vi "GetThermAlarmAnalogInputUnitsValue.vi"(8 "error in":errorcluster, 10 "ThermAlarm number":T1=1 items=["ThermAlarm 1"=1, "ThermAlarm 2"=2, "ThermAlarm 3"=3, "ThermAlarm 4"=4], 11 "VISA resource name":refnum<visa-resource-name>) -> (0 "error out":errorcluster, 2 "ThermAlarm analog input units value":string, 3 "VISA resource name out":refnum<visa-resource-name>)   [LabVIEW 2023, in "Thermotron 8800.lvlib"]
doc: "AACH\nCommand name: Therm-Alarm analog input value\nCommand name: Send Therm-Alarm analog input units value\nCommand type: System status\nDescription: The 8800 returns 1-3 characters for the value. Common unit codes are % and T (torr).\nSyntax: AACHn?\nWhere n is a Therm-Alarm number (1 to 4).\nData type: 1-3 characters\nQuery example: AACH1?\n8800 response: T (The analog input of Therm-Alarm 1 is programmed in torr.)"
uses:
  Thermotron 8800.lvlib
  Private/ThermAlarmNumber.ctl
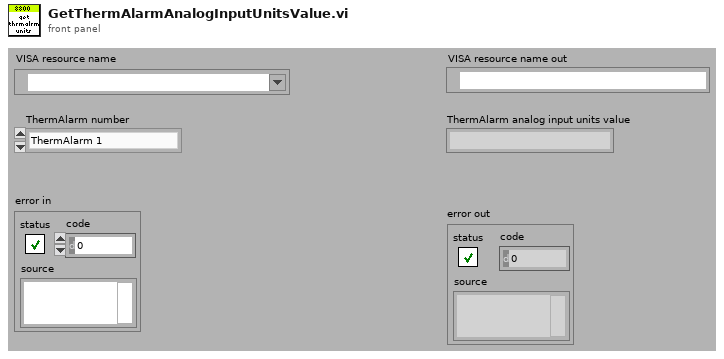
[diagram p1: front panel]
types:
  T1 = typedef "Thermotron 8800.lvlib/ThermAlarmNumber.ctl" = u16
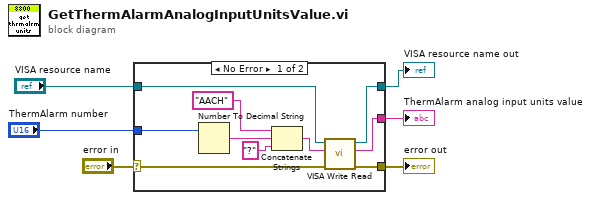
[diagram p0: block diagram]
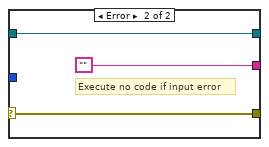
[diagram p2: hidden frame]
diagram:
  n1 = case shown="No Error" "error in" {
    selector: "error in" -> [w10 w19]
    tunnel: [w9 w19] -> w3
    tunnel: "VISA resource name" -> [w12 w18]
    tunnel: [w11 w18] -> w4
    tunnel: "ThermAlarm number" -> [w8 _]
    tunnel: [w7 ""] -> w1
    frame No Error {
      n2 = Number To Decimal String(number=w8) -> (decimal integer string=w16:string)  [unwired: 1 in]
      n3 = Concatenate Strings("AACH" ("8800 Command"), w16, "?" ("8800 Command")) -> (w15:string)
      n4 = call "VISA Write Read.vi"("error in (no error)"=w10, "8800 Command"=w15, "VISA Refnum in"=w12) -> ("error out"=w9:errorcluster, "read buffer"=w7:string, "VISA Refnum out"=w11:refnum<visa-resource-name>)  [unwired: 6 in]
    }
    frame Error {
      # "Execute no code if input error"
    }
  }
  "error out" <- w3
  "VISA resource name out" <- w4
  "ThermAlarm analog input units value" <- w1
